vi "Get Waveform.vi"(11 "index":u32) -> (3 "waveform":picture)   [LabVIEW 2020]
doc: "Returns an image of the waveform selected by index (0..4)."
uses:
  sub VIs/Globals.vi
panel:
  out "Waveform Graph":dbl[](graph)
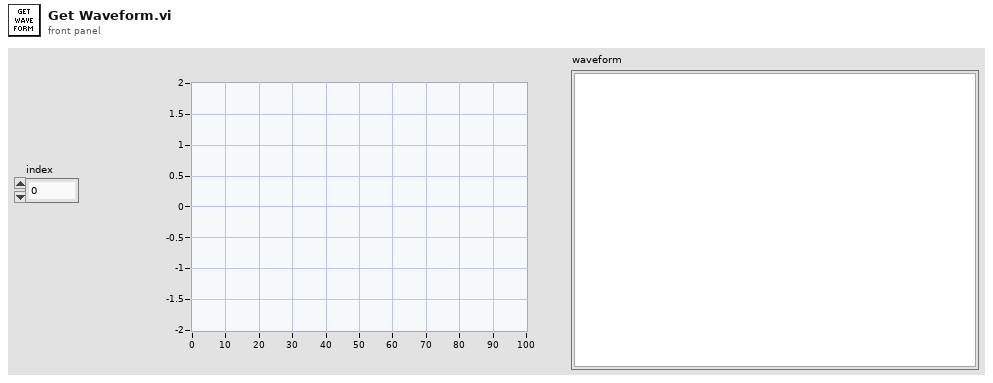
[diagram p1: front panel]
types:
  T1 = typedef "imagedata.ctl" = cluster{"image type":i32, "image depth":i32, "image":u8[], "mask":u8[], "colors":u32[], "Rectangle":cluster{"left":i16, "top":i16, "right":i16, "bottom":i16}}
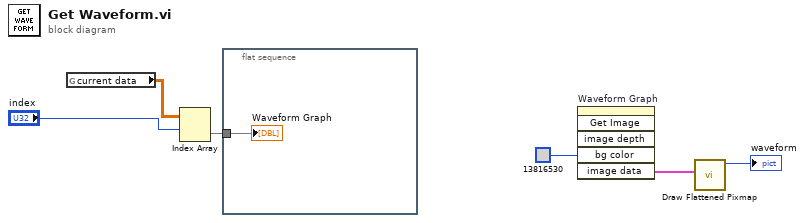
[diagram p0: block diagram]
diagram:
  n1 = global read "Globals.vi" "current data"() -> (w6:dbl[][])
  n2 = Index Array(array=w6, index (row)="index") -> (element=w4:dbl[])  [unwired: 1 in]
  n3 = flat-sequence {
    tunnel: w4 -> [w7]
    frame #0 {
      "Waveform Graph" <- w7
    }
  }
  n4 = invoke on="Waveform Graph" class="WFGraph (strict)" method="Get Image"("bg color"=u32 13816530 ("Background Color")) -> ("image data"=w2:T1)  [unwired: 5 in, 5 out]
  n5 = call <vilib>:"Draw Flattened Pixmap.vi"("image data"=w2) -> ("new picture"=→"waveform":picture)  [unwired: 8 in]
